vi "LVSWrt_Rd.vi"(6 "delay":u32=10, 9 "WriteBuf":string="?", 11 "COM Port":refnum<visa-resource-name>) -> (0 "ComError":bool, 2 "string read":string)   [LabVIEW 2013]
uses:
  instr.lib/lvserial/lvserial.lvlib
  <vilib>/Utility/error.llb/DialogType.ctl
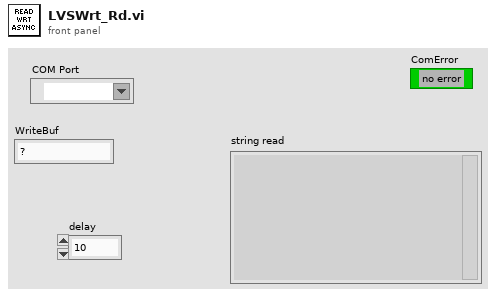
[diagram p1: front panel]
types:
  T1 = typedef "DialogType.ctl" = u16
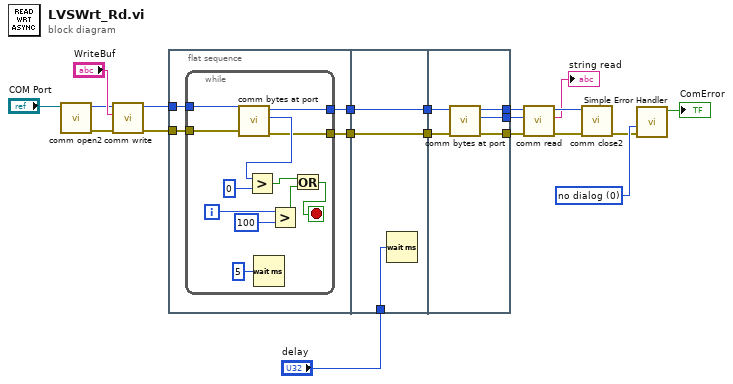
[diagram p0: block diagram]
diagram:
  w8 = T1 0 items=["no dialog", "OK message", "continue or stop message", "OK message + warnings", "continue/stop + warnings"] ("type of dialog (OK msg:1)")
  n1 = call "comm open2.vi"("Comm Port Name"="COM Port") -> ("error out"=w9:errorcluster, "Comm Handle"=w10:u32)  [unwired: 4 in, 1 out]
  n2 = call "comm write.vi"("error in (no error)"=w9, "string to write"="WriteBuf", "Comm Handle"=w10) -> ("error out"=w11:errorcluster, "dup Comm Handle"=w12:u32)  [unwired: 6 in, 1 out]
  n3 = flat-sequence {
    tunnel: w12 -> [w24]
    tunnel: w11 -> [w23]
    tunnel: [w22] -> w5
    tunnel: [w21] -> w3
    tunnel: w5 -> [w39]
    tunnel: [w39] -> w4
    tunnel: w3 -> [w38]
    tunnel: [w38] -> w2
    tunnel: "delay" -> [w37]
    tunnel: [w44] -> w16
    tunnel: w4 -> [w43]
    tunnel: w2 -> [w42]
    tunnel: [w41] -> w14
    tunnel: [w40] -> w13
    frame #0 {
      n4 = while {
        tunnel: w24 -> [w28]
        tunnel: w23 -> [w27]
        tunnel: [w26] -> w22
        tunnel: [w25] -> w21
        i -> [w29]
        stop <- w31 stop-if-true
        n5 = call "comm bytes at port.vi"("error in (no error)"=w27, "Comm Handle"=w28) -> ("error out"=w25:errorcluster, "bytes at port"=w30:u32, "dup Comm Handle"=w26:u32)  [unwired: 7 in]
        n6 = Greater?(x=w30, y=u32 0) -> (0:w34:bool)
        n7 = Wait (ms)(milliseconds to wait=u32 5) -> ()  [unwired: 1 out]
        n8 = Greater?(x=w29, y=100) -> (0:w35:bool)
        n9 = Or(x=w34, y=w35) -> (x .or. y?=w31:bool)
      }
    }
    frame #1 {
      n10 = Wait (ms)(milliseconds to wait=w37) -> ()  [unwired: 1 out]
    }
    frame #2 {
      n11 = call "comm bytes at port.vi"("error in (no error)"=w42, "Comm Handle"=w43) -> ("error out"=w40:errorcluster, "bytes at port"=w44:u32, "dup Comm Handle"=w41:u32)  [unwired: 7 in]
    }
  }
  n12 = call "comm read.vi"("error in (no error)"=w13, "requested byte count"=w16, "Comm Handle"=w14) -> ("error out"=w15:errorcluster, "string read"=→"string read":string, "dup Comm Handle"=w19:u32)  [unwired: 5 in, 1 out]
  n13 = call "comm close2.vi"("error in (no error)"=w15, "Comm Handle"=w19) -> ("error out"=w6:errorcluster)  [unwired: 5 in]
  n14 = call <vilib>:"Simple Error Handler.vi"("type of dialog (OK msg:1)"=w8, "error in (no error)"=w6) -> ("error?"=→"ComError":bool)  [unwired: 7 out]
